vi "Energize.vi"(8 "error in (no error)":errorcluster, 11 "CIFCorePlugin in":refnum<class "CIFCorePlugin.lvclass">) -> (0 "error out":errorcluster, 3 "CIFCorePlugin out":refnum<class "CIFCorePlugin.lvclass">)   [LabVIEW 2021, in "CIFCorePlugin.lvclass"]
uses:
  CIFCorePlugin.lvclass
  CIFCorePlugin.lvclass/CIFCorePlugin.ctl
  CIFUtilities/CIFClocks/Core/Get Time.vi
  CIFUtilities/CIFClocks/Time Conversion/LabVIEW Time to UTC Time.vi
  CIFUtilities/CIFClocks/SubVIs/Add Error.vi
  <vilib>/Platform/TimedLoop/XDataNode/XDataNode.xnode
  <vilib>/Platform/TimedLoop/XDataNode/nitl_modes.ctl
  <vilib>/Platform/TimedLoop/XDataNode/XDNodeRunTimeDep.lvlib
  <vilib>/Platform/TimedLoop/XDataNode/wakeup.ctl
  <vilib>/Platform/TimedLoop/XDataNode/timing_clust.ctl
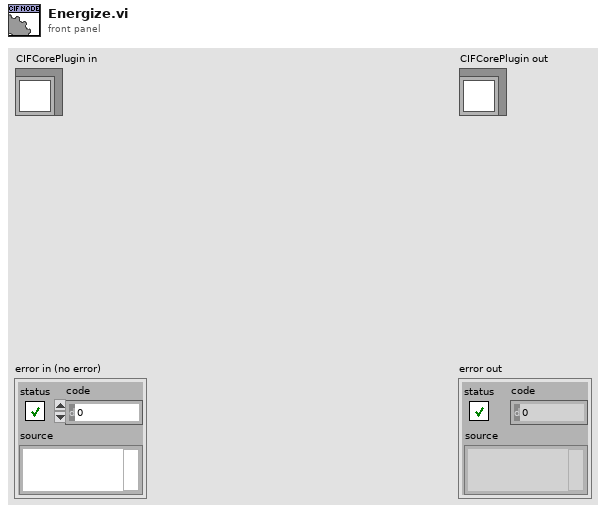
[diagram p1: front panel]
types:
  T1 = typedef "XDNodeRunTimeDep.lvlib/timing_clust.ctl" = cluster{"Expected End [f-1]":u64, "Actual End [f-1]":u64, "Finished Late? [f-1]":bool, "Expected End [i-1]":u64, "Actual End [i-1]":u64, "Finished Late? [i-1]":bool, "Expected Start [i]":u64, "Actual Start [i]":u64, "Expected Start [f]":u64, "Actual Start [f]":u64, "Source Name":string, "Structure Name":string, "Period":i64, "Deadline":i64, "Offset":i64, "Start":i64, "Priority":i32, "Timeout":i32, "Mode":T2, "Wakeup Reason":T3, "Error":errorcluster, "Source Type":string, "Secondary Source Type":string, "Global End Time":u64, "Global Start Time":u64, "Frame Duration":u64, "Iteration Duration":u64, "Assigned CPU":i32, "I/O Scan Engine Mode":u32}
  T2 = typedef "XDNodeRunTimeDep.lvlib/nitl_modes.ctl" = enum32{"No Change", "Process missed periods, maintain original phase", "Discard missed periods, maintain original phase", "Process missed periods, ignore original phase", "Discard missed periods, ignore original phase"}
  T3 = typedef "XDNodeRunTimeDep.lvlib/wakeup.ctl" = enum32{"Normal", "Aborted", "Asynchronous wakeup", "Timing source error", "Timed loop error", "Timeout"}
  T4 = typedef "CIFCorePlugin.lvclass/Prepare State Logic.ctl" = enum16{"Listen", "Prepare", "Error", "Destroy"}
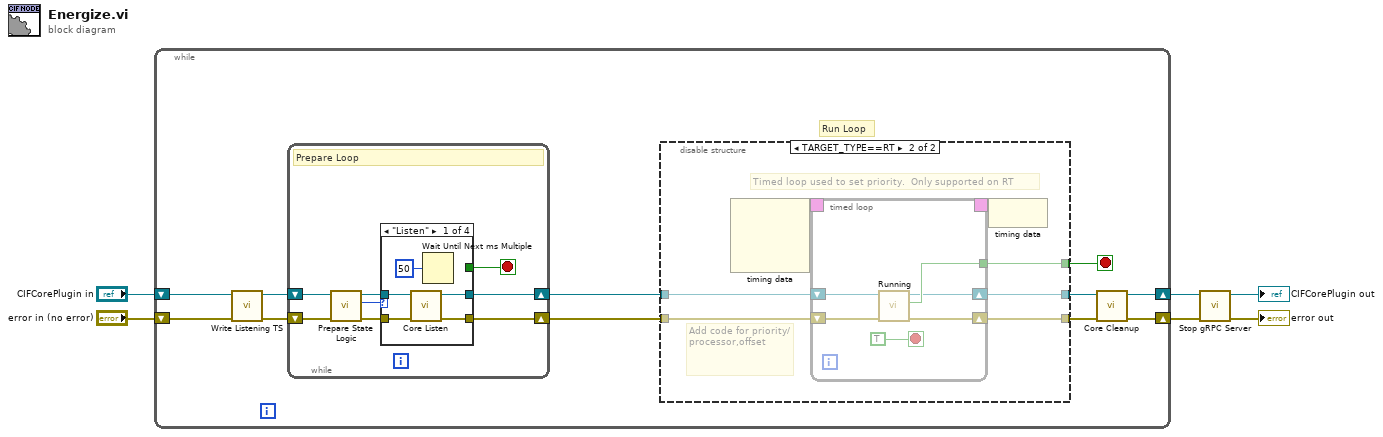
[diagram p0: block diagram]
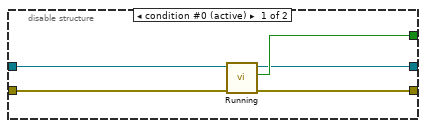
[diagram p2: hidden frame]
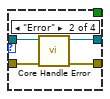
[diagram p3: hidden frame]
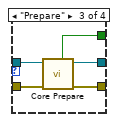
[diagram p4: hidden frame]
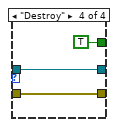
[diagram p5: hidden frame]
diagram:
  n1 = while {
    shift-right: [w14] -> w4
    shift-left: "CIFCorePlugin in" -> [w12]
    shift-right: [w13] -> w3
    shift-left: "error in (no error)" -> [w11]
    stop <- w17 stop-if-true
    # "Run Loop"
    n2 = call "Write Listening TS.vi"("error in (no error)"=w11, "CIFCorePlugin in"=w12) -> ("error out"=w9:errorcluster, "CIFCorePlugin out"=w10:refnum<class "CIFCorePlugin.lvclass">)  [unwired: 8 in]
    n3 = while {
      shift-right: [w47] -> w8
      shift-left: w10 -> [w40]
      shift-right: [w42] -> w7
      shift-left: w9 -> [w43]
      stop <- w41 stop-if-true
      # "Prepare Loop"
      n4 = call "Prepare State Logic.vi"("error in (no error)"=w43, "CIFCorePlugin in"=w40) -> ("error out"=w44:errorcluster, "Prepare State Logic"=w45:T4, "CIFCorePlugin out"=w46:refnum<class "CIFCorePlugin.lvclass">)  [unwired: 7 in]
      n5 = case shown="\"Listen\"" w45 {
        tunnel: [w49 w56 w61 w64] -> w47
        tunnel: w46 -> [w52 w53 w57 w64]
        tunnel: w44 -> [w51 w54 w58 w63]
        tunnel: [w50 w55 w60 w63] -> w42
        tunnel: [_ _ w59 TRUE ("Transition to Run")] -> w41
        frame "Listen" {
          n6 = call "Core Listen.vi"("error in (no error)"=w51, "CIFTemplateNode in"=w52) -> ("error out"=w50:errorcluster, "CIFTemplateNode out"=w49:refnum<class "CIFCorePlugin.lvclass">)  [unwired: 8 in]
          n7 = Wait Until Next ms Multiple(millisecond multiple=u32 50) -> ()  [unwired: 1 out]
        }
        frame "Error" {
          n8 = call "Core Handle Error.vi"("error in (no error)"=w54, "CIFTemplateNode in"=w53) -> ("error out"=w55:errorcluster, "CIFTemplateNode out"=w56:refnum<class "CIFCorePlugin.lvclass">)  [unwired: 8 in]
        }
        frame "Prepare" {
          n9 = call "Core Prepare.vi"("error in (no error)"=w58, "CIFTemplateNode in"=w57) -> ("error out"=w60:errorcluster, "CIFTemplateNode out"=w61:refnum<class "CIFCorePlugin.lvclass">, "Transition to Run"=w59:bool)  [unwired: 7 in]
        }
        frame "Destroy" {
        }
      }
    }
    n10 = disable-structure shown="TARGET_TYPE==RT" {
      disable-tunnel: w8 -> [w22 w27]
      disable-tunnel: w7 -> [w21 w26]
      disable-tunnel: [w20 w25] -> w17
      disable-tunnel: [w19 w24] -> w16
      disable-tunnel: [w18 w23] -> w15
      frame condition #0 (active) {
        n11 = call "Running.vi"("error in (no error)"=w21, "CIFCorePlugin in"=w22) -> ("error out"=w18:errorcluster, "Destroy"=w20:bool, "CIFCorePlugin out"=w19:refnum<class "CIFCorePlugin.lvclass">)  [unwired: 7 in]
      }
      frame condition #1 {
        # "Add code for priority/processor,offset"
        # "Timed loop used to set priority.  Only supported on RT"
        n12 = node-c288() -> (w29:T1)  [unwired: 3 in]
        n13 = timed-loop {
          timing: w29 -> [_]
          timing-out: [_] -> w28
          shift-right: [w33] -> w24
          shift-left: w27 -> [w31]
          shift-right: [w32] -> w23
          shift-left: w26 -> [w30]
          tunnel: [w34] -> w25
          stop <- TRUE stop-if-true
          n14 = call "Running.vi"("error in (no error)"=w30, "CIFCorePlugin in"=w31) -> ("error out"=w32:errorcluster, "Destroy"=w34:bool, "CIFCorePlugin out"=w33:refnum<class "CIFCorePlugin.lvclass">)  [unwired: 7 in]
        }
        n15 = node-c288(w28) -> ()
      }
    }
    n16 = call "Core Cleanup.vi"("error in (no error)"=w15, "CIFTemplateNode in"=w16) -> ("error out"=w13:errorcluster, "CIFTemplateNode out"=w14:refnum<class "CIFCorePlugin.lvclass">)  [unwired: 8 in]
  }
  n17 = call "Stop gRPC Server.vi"("error in (no error)"=w3, "CIFCorePlugin in"=w4) -> ("error out"=→"error out":errorcluster, "CIFCorePlugin out"=→"CIFCorePlugin out":refnum<class "CIFCorePlugin.lvclass">)  [unwired: 8 in]
